vi "Untitled 4.vi"() -> ()   [LabVIEW 2025]
panel:
  out "subarray":string[](array[string])
  in  "Multicolumn Listbox":i32(listbox)
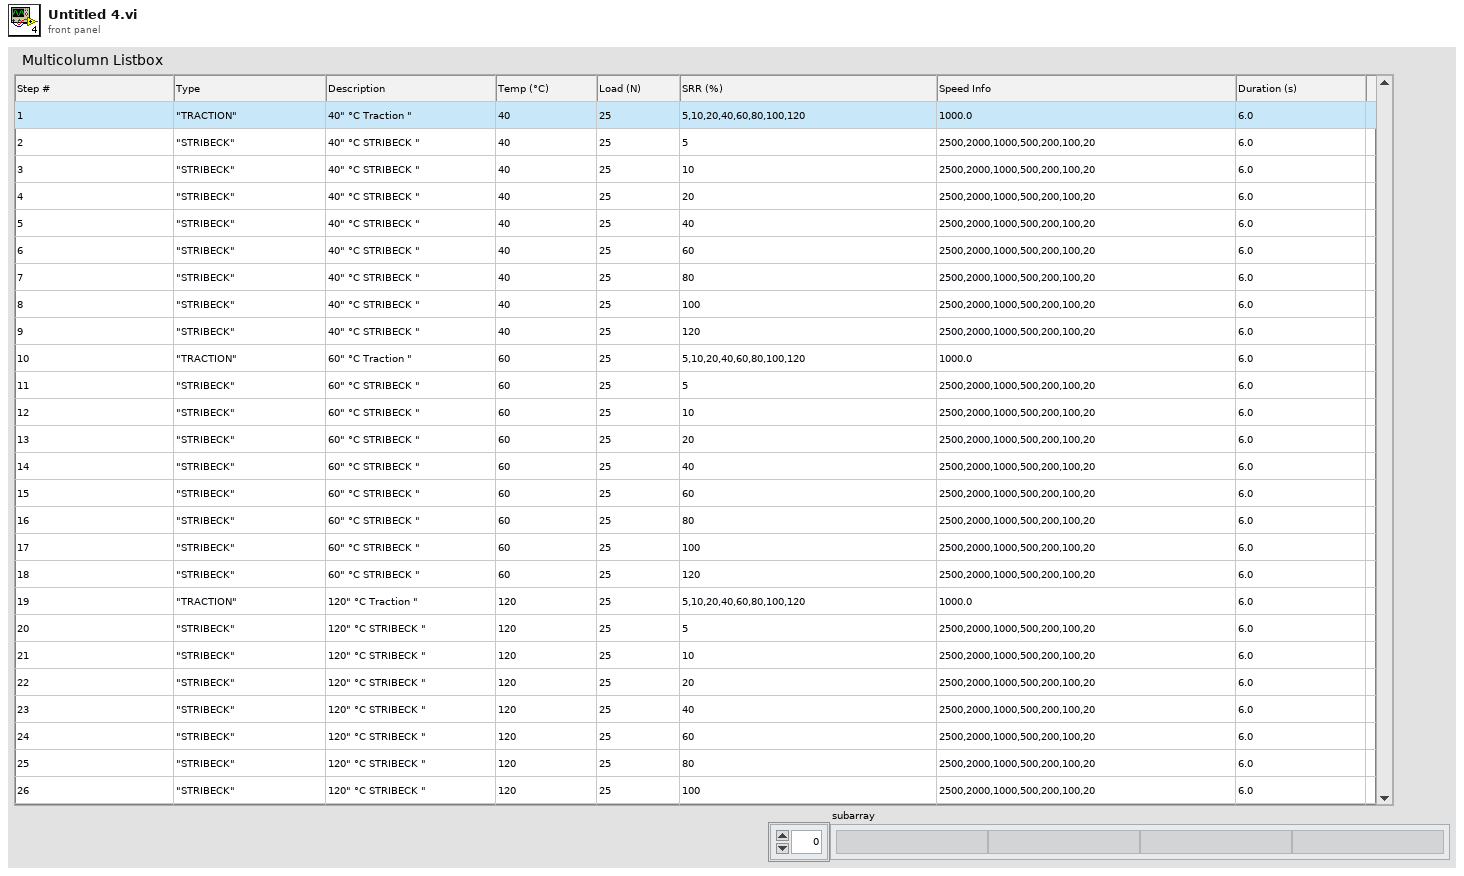
[diagram p1: front panel]
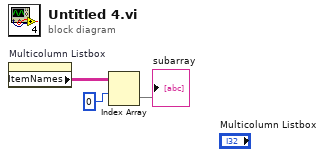
[diagram p0: block diagram]
diagram:
  n1 = property on="Multicolumn Listbox" class="MCListbox (strict)"() -> ("ItemNames"=w3:string[][])  [unwired: 2 in, 2 out]
  n2 = Index Array(array=w3, index (row)=0 ("disabled index (col)")) -> (element=→"subarray":string[])  [unwired: 1 in]
